vi "Receive Signal DBL.vi"(8 "error in":errorcluster, 10 "Signal Name":string, 11 "DBC Communication in":refnum<class "DBC Communication.lvclass">) -> (0 "error out":errorcluster, 1 "Time Stamp":timestamp format="%<%x %.3X>T", 2 "Value":dbl, 3 "DBC Communication out":refnum<class "DBC Communication.lvclass">)   [LabVIEW 2024, in "DBC Communication.lvclass"]
uses:
  DBC Communication.lvclass
  DBC Communication.lvclass/DBC Communication.ctl
  <vilib>/xnet/xnet.llb/XNET Frame Type CAN.ctl
  <vilib>/Utility/miscctls.llb/LVMapReplaceAction.ctl
  c9a96274-a027-4ccf-b481-50e0b552ac68.vi
  <vilib>/Utility/error.llb/Trim Whitespace One-Sided.vi
  c9a96274-a027-4ccf-b481-50e0b552ac68.vi/d4db2432-cc9c-482c-8957-dac855435ef6.vi
  c9a96274-a027-4ccf-b481-50e0b552ac68.vi/86fbf154-bd7b-49a2-8ab2-a837b2a95f24.vi
  c9a96274-a027-4ccf-b481-50e0b552ac68.vi/3b95b01e-1ec2-4565-bcd9-7606a5281010.vi
  c9a96274-a027-4ccf-b481-50e0b552ac68.vi/96a08935-737a-44b2-979c-a81d56408f7e.vi
  c9a96274-a027-4ccf-b481-50e0b552ac68.vi/d4db2432-cc9c-482c-8957-dac855435ef6.vi/6eaecd13-6e48-4772-a921-b51ebdf84d88.vi
  c9a96274-a027-4ccf-b481-50e0b552ac68.vi/d4db2432-cc9c-482c-8957-dac855435ef6.vi/d2d5f2b7-06f4-47f6-971c-049c3fdbb653.vi
  c9a96274-a027-4ccf-b481-50e0b552ac68.vi/3b95b01e-1ec2-4565-bcd9-7606a5281010.vi/6eaecd13-6e48-4772-a921-b51ebdf84d88.vi
  c9a96274-a027-4ccf-b481-50e0b552ac68.vi/3b95b01e-1ec2-4565-bcd9-7606a5281010.vi/d2d5f2b7-06f4-47f6-971c-049c3fdbb653.vi
  c9a96274-a027-4ccf-b481-50e0b552ac68.vi/96a08935-737a-44b2-979c-a81d56408f7e.vi/6eaecd13-6e48-4772-a921-b51ebdf84d88.vi
  c9a96274-a027-4ccf-b481-50e0b552ac68.vi/96a08935-737a-44b2-979c-a81d56408f7e.vi/d2d5f2b7-06f4-47f6-971c-049c3fdbb653.vi
  <vilib>/xnet/xnet.llb/XNET Convert (Frame CAN to Signal).vi
  <vilib>/Comparison/Less/Less Functor/Less Functor.lvclass
  Interfaces/ICommunicate/ICommunicate.lvclass
  Interfaces/IMessage/IMessage.lvclass
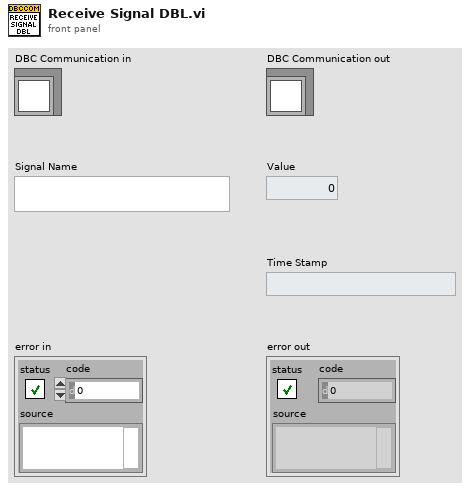
[diagram p1: front panel]
types:
  T1 = typedef "LVMapReplaceAction.ctl" = enum32{"Modify Entry only if found", "Add or Modify Entry", "Delete Entry"}
  T2 = typedef "XNET Frame Type CAN.ctl" = u8
  T3 = cluster{"timestamp":timestamp, "payload":u8[], "identifier":u32, "type":T2, "extended?":bool, "echo?":bool}
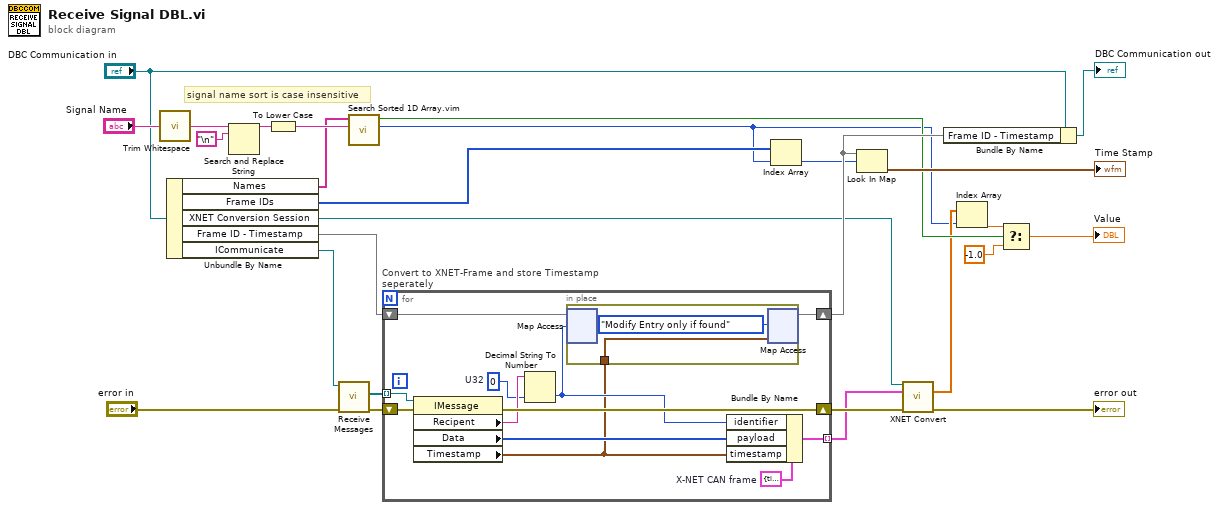
[diagram p0: block diagram]
diagram:
  # "signal name sort is case insensitive"
  n1 = call <vilib>:"Trim Whitespace.vi"("string"="Signal Name") -> ("trimmed string"=w3:string)  [unwired: 1 in]
  n2 = Unbundle By Name("DBC Communication in") -> ("Names"=w1:string[], "Frame IDs"=w6:u32[], "XNET Conversion Session"=w15:refnum<k21>, "Frame ID - Timestamp"=w21:map{u32, timestamp}, "ICommunicate"=w22:refnum<class "ICommunicate.lvclass">)
  n3 = Search and Replace String(input string=w3, search string="\n") -> (result string=w18:string)  [unwired: 6 in, 3 out]
  n4 = To Lower Case(string=w18) -> (all lower case string=w2:string)
  n5 = call-dynamic "Receive Messages.vi"("error in"="error in", "ICommunicate in"=w22) -> ("error out"=w13:errorcluster, "Messages"=w14:refnum<class "IMessage.lvclass">[])  [unwired: 7 in, 1 out]
  n6 = call "Search Sorted 1D Array.vim"("element"=w2, "sorted 1D array"=w1) -> ("nearest index"=w5:i32, "found?"=w10:bool)  [unwired: 8 in]
  n7 = for "Convert to XNET-Frame and store Timestamp seperately" {
    tunnel: w14 -> [w34] mode=indexing
    shift-right: [w37] -> w12
    shift-left: w13 -> [w33]
    tunnel: [w36] -> w11 mode=indexing
    shift-right: [w28] -> w17
    shift-left: w21 -> [w32]
    w29 = u32 0  # U32
    w39 = T3 {"timestamp"=timestamp(0 s since 1904-01-01), "payload"=[], "identifier"=0, "type"=0, "extended?"=FALSE, "echo?"=FALSE}  # X-NET CAN frame
    n8 = property class="IMessage"(reference=w34, error in=w33) -> (error out=w37:errorcluster, "Recipent"=w35:string, "Data"=w38:u8[], "Timestamp"=w30:timestamp)  [unwired: 1 out]
    n9 = Decimal String To Number(string=w35, default (0L)=w29) -> (number=w31:u32)  [unwired: 1 in, 1 out]
    n10 = in-place {
      in-place-border: w30 -> [w41]
      n11 = in-place-map #1(w32, w31) -> ()  [unwired: 1 in, 2 out]
      n12 = in-place-map #1(w41, LVMapReplaceAction."Modify Entry only if found" ("action")) -> (w28:map{u32, timestamp})  [unwired: 2 out]
    }
    n13 = Bundle By Name(cluster=w39, "identifier"=w31, "payload"=w38, "timestamp"=w30) -> (w36:T3)
  }
  n14 = Index Array(array=w6, index=w5) -> (element=w4:u32)
  n15 = Look In Map(map=w17, key=w4) -> (value=→"Time Stamp":timestamp)  [unwired: 1 in, 1 out]
  n16 = call-poly <vilib>:"XNET Convert.vi"("session in"=w15, "frame data"=w11, "error in (no error)"=w12) -> ("signal data"=w7:dbl[], "error out"=→"error out":errorcluster)  [unwired: 10 in, 1 out]
  n17 = Bundle By Name(cluster="DBC Communication in", "Frame ID - Timestamp"=w17) -> (→"DBC Communication out":refnum<class "DBC Communication.lvclass">)
  n18 = Index Array(array=w7, index=w5) -> (element=w9:dbl)
  n19 = Select(t=w9, s=w10, f=-1.0) -> (s? t:f=→"Value":dbl)
